vi "Insert Start Message.vi"(8 "error in (no error)":errorcluster, 10 "Start Time":timestamp, 11 "BehaviorData in":refnum<class "BehaviorData.lvclass">) -> (0 "error out":errorcluster, 3 "BehaviorData out":refnum<class "BehaviorData.lvclass">)   [LabVIEW 2014, in "BehaviorData.lvclass"]
uses:
  BehaviorData.lvclass
  Database/BehPrimary.ctl
  AcquireTraces/AcquireTraces.lvclass
  AcquistionObject/AcquistionObject.lvclass
panel:
  out "BehPK":T1
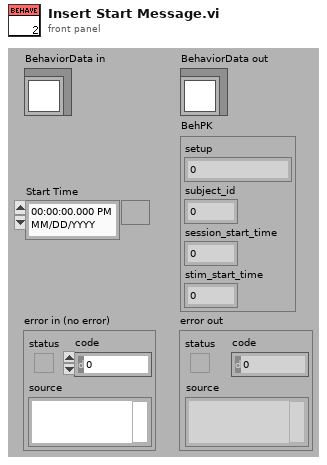
[diagram p1: front panel]
types:
  T1 = typedef "BehPrimary.ctl" = cluster{"setup":u8, "subject_id":i32, "session_start_time":dbl, "stim_start_time":dbl}
  T2 = cluster{"setup":u8, "subject_id":i32, "session_start_time":dbl, "stim_start_time":dbl, "beh_start_time":dbl, "beh_path":path, "beh_traces_type":string, "beh_stop_time":dbl}
  T3 = typedef "NI_Database_API.lvlib/Conn ObjectReference.ctl" = refnum<k1>
  T4 = cluster{"reference":T3, "table":string, "columns":string[], i32}
  T5 = cluster{cluster{"reference":T3, "table":string, "columns":string[], i32}, "Variant":variant}
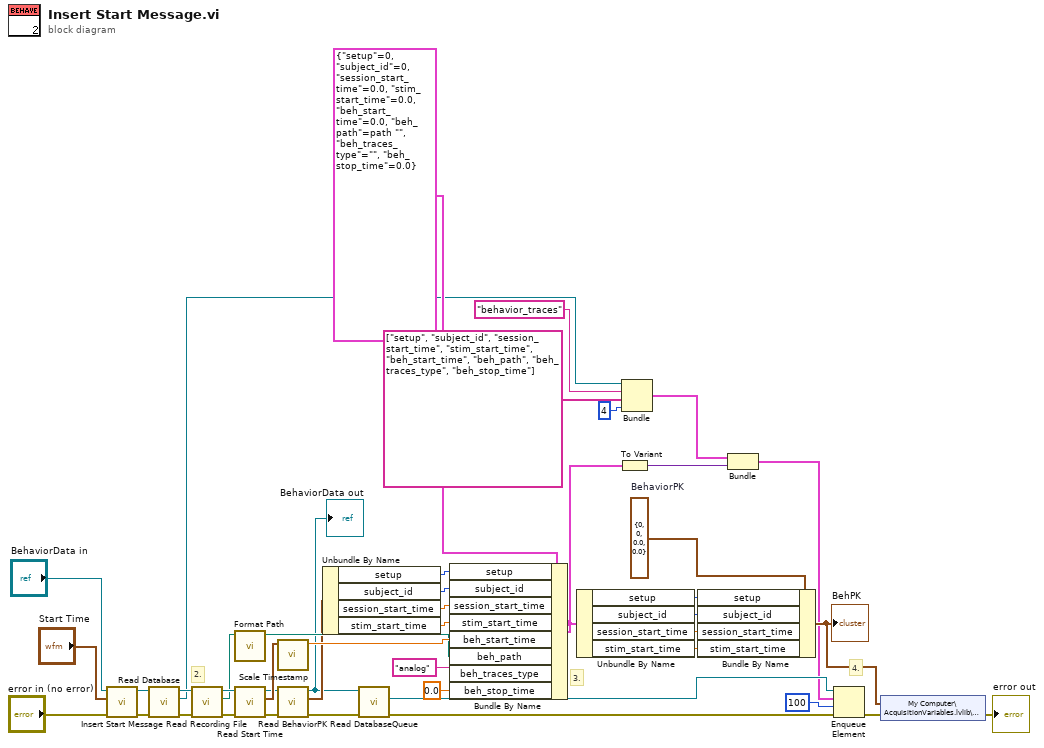
[diagram p0: block diagram]
diagram:
  w31 = T1 {"setup"=0, "subject_id"=0, "session_start_time"=0.0, "stim_start_time"=0.0}  # BehaviorPK
  # "4."
  # "2."
  # "3."
  n1 = call-parent "Insert Start Message.vi"("error in (no error)"="error in (no error)", "Start Time"="Start Time", "AcquireTraces in"="BehaviorData in") -> ("error out"=w27:errorcluster, "AcquireTraces out"=w28:refnum<class "BehaviorData.lvclass">)  [unwired: 7 in]
  n2 = call-dynamic "Read Database.vi"("error in (no error)"=w27, "AcquistionObject in"=w28) -> ("error out"=w30:errorcluster, "reference"=w12:T3, "AcquistionObject out"=w29:refnum<class "BehaviorData.lvclass">)  [unwired: 7 in]
  n3 = call-dynamic "Read Recording File.vi"("error in (no error)"=w30, "AcquistionObject in"=w29) -> ("error out"=w34:errorcluster, "Recording File"=w20:path, "AcquistionObject out"=w35:refnum<class "BehaviorData.lvclass">)  [unwired: 7 in]
  n4 = call "Format Path.vi"("Input path"=w20) -> ("Output path"=w19:path)  [unwired: 10 in]
  n5 = call-dynamic "Read Start Time.vi"("error in (no error)"=w34, "AcquistionObject in"=w35) -> ("error out"=w18:errorcluster, "Start Time"=w24:timestamp, "AcquistionObject out"=w17:refnum<class "BehaviorData.lvclass">)  [unwired: 7 in]
  n6 = call "Scale Timestamp.vi"("Time Stamp"=w24) -> ("Scaled timestamp"=w23:dbl)  [unwired: 10 in]
  n7 = call-dynamic "Read BehaviorPK.vi"("error in (no error)"=w18, "BehaviorData in"=w17) -> ("error out"=w6:errorcluster, "BehaviorPK"=w16:T1, "BehaviorData out"=w2:refnum<class "BehaviorData.lvclass">)  [unwired: 7 in]
  "BehaviorData out" <- w2
  n8 = Unbundle By Name(w16) -> ("setup"=w41:u8, "subject_id"=w40:i32, "session_start_time"=w21:dbl, "stim_start_time"=w26:dbl)
  n9 = call-dynamic "Read DatabaseQueue.vi"("error in (no error)"=w6, "AcquistionObject in"=w2) -> ("error out"=w7:errorcluster, "DatabaseQueue"=w5:refnum<queue>)  [unwired: 7 in, 1 out]
  n10 = Bundle By Name(cluster=T2 {"setup"=0, "subject_id"=0, "session_start_time"=0.0, "stim_start_time"=0.0, "beh_start_time"=0.0, "beh_path"=path "", "beh_traces_type"="", "beh_stop_time"=0.0} ("Cluster"), "setup"=w41, "subject_id"=w40, "session_start_time"=w21, "stim_start_time"=w26, "beh_start_time"=w23, "beh_path"=w19, "beh_traces_type"="analog", "beh_stop_time"=0.0) -> (w9:T2)
  n11 = Unbundle By Name(w9) -> ("setup"=w39:u8, "subject_id"=w38:i32, "session_start_time"=w37:dbl, "stim_start_time"=w22:dbl)
  n12 = To Variant(anything=w9) -> (Variant=w13:variant)
  n13 = Bundle("reference"=w12, "table"="behavior_traces", "columns"=string[] ["setup", "subject_id", "session_start_time", "stim_start_time", "beh_start_time", "beh_path", "beh_traces_type", "beh_stop_time"], 4) -> (w14:T4)  [unwired: 1 in]
  n14 = Bundle By Name(cluster=w31, "setup"=w39, "subject_id"=w38, "session_start_time"=w37, "stim_start_time"=w22) -> (w36:T1)
  "BehPK" <- w36
  n15 = Bundle(w14, "Variant"=w13) -> (w4:T5)  [unwired: 1 in]
  n16 = Enqueue Element(queue=w5, element=w4, timeout in ms (-1)=100, error in (no error)=w7) -> (error out=w3:errorcluster)  [unwired: 2 out]
  n17 = shared-variable "My Computer\\AcquisitionVariables.lvlib\\BehaviorPK"(w36, error in=w3) -> (error out=→"error out":errorcluster)
